vi "subscribeTelemetry.vi"(8 "error in (no error)":errorcluster, 11 "SAL_Listener in":refnum<class "SAL_Listener.lvclass">) -> (0 "error out":errorcluster, 3 "SAL_Listener out":refnum<class "SAL_Listener.lvclass">)   [LabVIEW 2015, in "SAL_Listener.lvclass"]
uses:
  SAL_Listener.lvclass
  SALLV_domeADB/SALLV_domeADB.lvlib
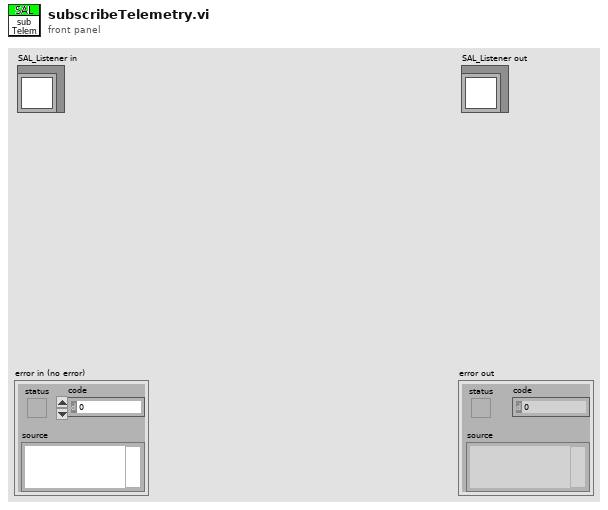
[diagram p1: front panel]
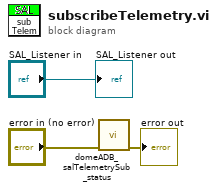
[diagram p0: block diagram]
diagram:
  n1 = call "domeADB_salTelemetrySub_status.vi"("error in (no error)"="error in (no error)") -> ("error out"=→"error out":errorcluster)  [unwired: 9 in, 1 out]
  "SAL_Listener out" <- "SAL_Listener in"
